vi "Constructor.vi"(8 "error in (no error)":errorcluster, 10 "Column Configuration":refnum<class "Basic Column Configuration.lvclass">, 11 "By-Value Column in":refnum<class "By-Value Column.lvclass">) -> (0 "error out":errorcluster, 3 "By-Value Column out":refnum<class "By-Value Column.lvclass">)   [LabVIEW 2020, in "Basic Columns.lvlib" / "By-Value Column.lvclass"]
uses:
  By-Value Column.lvclass
  Basic Columns/Column Configuration/Basic Column Configuration Class/Basic Column Configuration.lvclass
  C:/Users/User/Desktop/Raman Program/Database OOP/source/Database OOP/Column Libraries/Column Interface/Column Configuration Interface Class/Column Configuration.lvclass
  By-Value Column.lvclass/By-Value Column.ctl
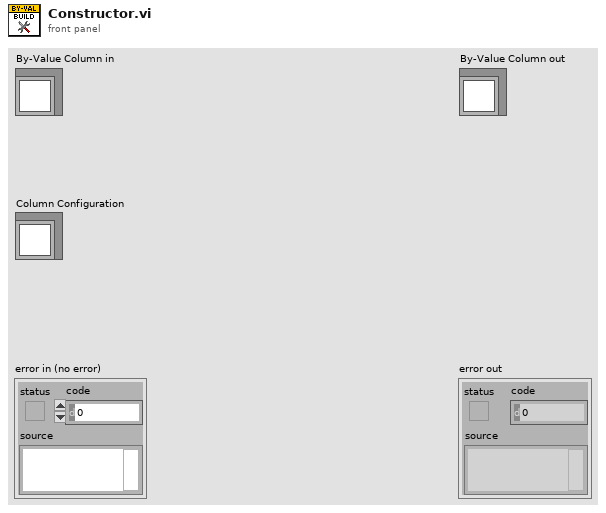
[diagram p1: front panel]
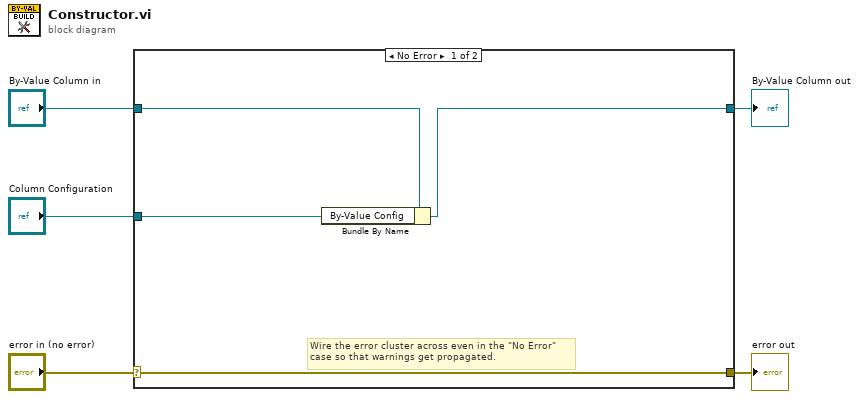
[diagram p0: block diagram]
diagram:
  n1 = case shown="No Error" "error in (no error)" {
    selector: "error in (no error)" -> [w9 w11]
    tunnel: [w9 w11] -> w4
    tunnel: [w6 w10] -> w2
    tunnel: "By-Value Column in" -> [w8 w10]
    tunnel: "Column Configuration" -> [w7 _]
    frame No Error {
      # "Wire the error cluster across even in the \"No Error\"\ncase so that warnings get propagated."
      n2 = Bundle By Name(cluster=w8, "By-Value Config"=w7) -> (w6:refnum<class "By-Value Column.lvclass">)
    }
    frame Error {
    }
  }
  "error out" <- w4
  "By-Value Column out" <- w2
